vi "Circle_Sub_VI.vi"(11 "Radius":dbl) -> (1 "Area":dbl, 2 "Circumferrence":dbl, 3 "Diameter":dbl)   [LabVIEW 2018]
doc: "Bhai tu bas radius daal, tera bhai yaha diameter,circumferrence aur area nikalega."
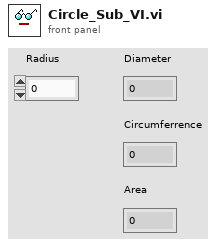
[diagram p1: front panel]
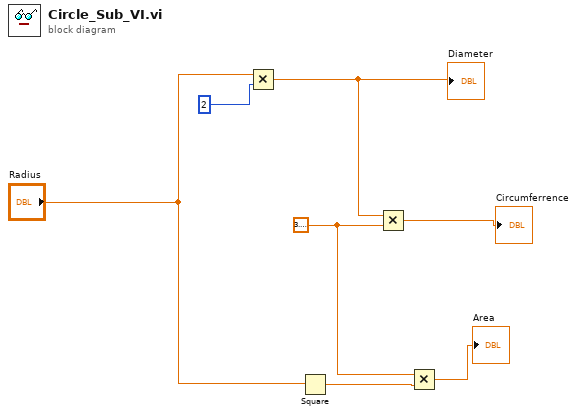
[diagram p0: block diagram]
diagram:
  w7 = 3.141592653589793
  n1 = Multiply(x="Radius", y=2) -> (x*y=w3:dbl)
  "Diameter" <- w3
  n2 = Square(x="Radius") -> (x^2=w6:dbl)
  n3 = Multiply(x=w3, y=w7) -> (x*y=→"Circumferrence":dbl)
  n4 = Multiply(x=w7, y=w6) -> (x*y=→"Area":dbl)
